vi "Lockstep Move (Polymorphic).vi"   [LabVIEW 2015, in "Zaber A Series.lvlib"]
doc: "Moves a lockstep group, which is a collection of axes that move in unison. You can specifiy the type of movement (absolute or relative) and the distance the device's native position units. See your device manual for the unit conversion, or use the Convert Position Units to Device Units VI to convert from standard length units.\n\nNo responses are returned with this VI, but if you would like to wait until the movement is completed to continue, you can combine this VI with the Poll Until Idle VI. \n\nThis VI requires that the Initialize VI has been called with the same serial port and that the lockstep group has been created with the Lockstep Enable VI. \n\nNote: See the Device Lookup control for the microstep size of your model, or check on the product specifications page for the product on www.zaber.com."
uses:
  Zaber A Series.lvlib
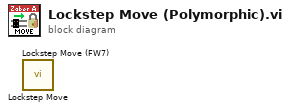
[diagram p0: block diagram]
diagram:
  n1 = call "Lockstep Move.vi"() -> ()  [unwired: 10 in, 2 out]
  n2 = call "Lockstep Move (FW7).vi"() -> ()  [unwired: 10 in, 2 out]
